vi "Error Handler - RT Loop - System Health and FPGA Monitoring.vi"(4 "FPGA Error (FPGA)":errorcluster caption="FPGA错误(FPGA)", 6 "Different Channel Count (FPGA)":bool caption="不同通道计数(FPGA)", 8 "error in (no error)":errorcluster caption="错误输入（无错误）", 9 "DMA FIFO Full (FPGA)":bool caption="DMA FIFO已满(FPGA)", 10 "Module Underflow (FPGA)":bool caption="模块下溢(FPGA)", 11 "Message Queue":refnum<queue> caption="消息队列") -> (3 "dup Message Queue":refnum<queue> caption="消息队列副本")   [LabVIEW 2013]
uses:
  support/Message Queue/Message Cluster.ctl
  support/Message Queue/Message Queue.lvlib
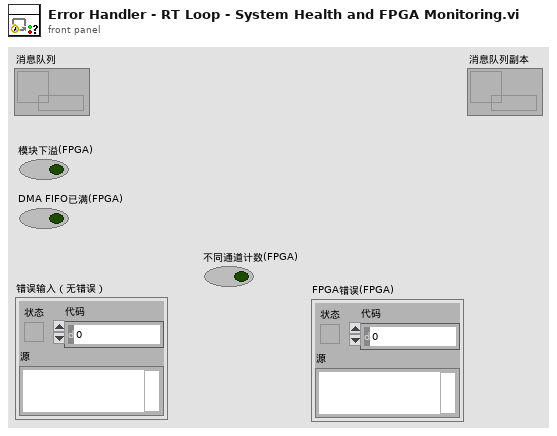
[diagram p1: front panel]
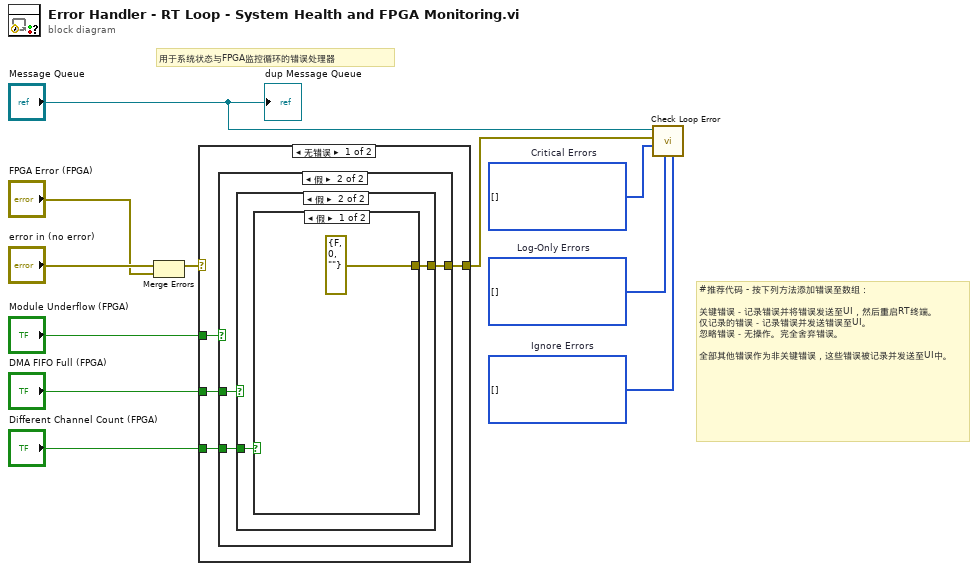
[diagram p0: block diagram]
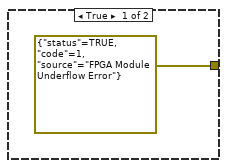
[diagram p2: hidden frame]
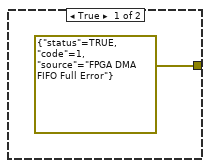
[diagram p3: hidden frame]
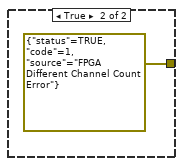
[diagram p4: hidden frame]
diagram:
  w9 = i32[] []  # Ignore Errors
  w10 = i32[] []  # Log-Only Errors
  w11 = i32[] []  # Critical Errors
  # "#推荐代码 - 按下列方法添加错误至数组：\n\n关键错误－记录错误并将错误发送至UI，然后重启RT终端。\n仅记录的错误－记录错误并发送错误至UI。\n忽略错误－无操作。完全舍弃错误。\n\n全部其他错误作为非关键错误，这些错误被记录并发送至UI中。"
  # "用于系统状态与FPGA监控循环的错误处理器"
  n1 = Merge Errors("error in (no error)", "FPGA Error (FPGA)") -> (w3:errorcluster)
  n2 = case shown="无错误" w3 {
    selector: w3 -> [_ w25]
    tunnel: "Module Underflow (FPGA)" -> [w15 _]
    tunnel: "DMA FIFO Full (FPGA)" -> [w13 _]
    tunnel: [w14 w25] -> w4
    tunnel: "Different Channel Count (FPGA)" -> [w12 _]
    frame No Error {
      n3 = case shown="假" w15 {
        tunnel: [errorcluster {"status"=TRUE, "code"=1, "source"="FPGA Module Underflow Error"} ("error constant") w19] -> w14
        tunnel: w13 -> [_ w18]
        tunnel: w12 -> [_ w17]
        frame True {
        }
        frame False {
          n4 = case shown="假" w18 {
            tunnel: [errorcluster {"status"=TRUE, "code"=1, "source"="FPGA DMA FIFO Full Error"} ("error constant") w22] -> w19
            tunnel: w17 -> [_ w21]
            frame True {
            }
            frame False {
              n5 = case shown="假" w21 {
                tunnel: [errorcluster {"status"=FALSE, "code"=0, "source"=""} ("error constant") errorcluster {"status"=TRUE, "code"=1, "source"="FPGA Different Channel Count Error"} ("error constant")] -> w22
                frame False {
                }
                frame True {
                }
              }
            }
          }
        }
      }
    }
    frame Error {
    }
  }
  n6 = call "Check Loop Error.vi"("Ignore Errors"=w9, "Log-Only Errors"=w10, "Critical Errors"=w11, "error to process"=w4, "Message Queue"="Message Queue") -> ()  [unwired: 5 in, 2 out]
  "dup Message Queue" <- "Message Queue"
